vi "Get Device Reference.vi"(11 "VeriStand Framework in":refnum<class "VeriStand DSF.lvclass">=refnum) -> (2 "Device Item Ref":T1=18446744073709551615 format="%.0x", 3 "VeriStand Framework out":refnum<class "VeriStand DSF.lvclass">)   [LabVIEW 2017, in "DSF Engine.lvlib" / "VeriStand DSF.lvclass"]
uses:
  VeriStand DSF.lvclass
  <vilib>/NI Veristand/Custom Device API/Custom Device Item Ref.ctl
  VeriStand DSF.lvclass/VeriStand DSF.ctl
  <vilib>/NI Veristand/Custom Device API/Custom Device API.lvlib
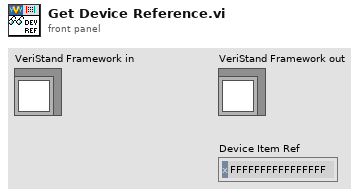
[diagram p1: front panel]
types:
  T1 = typedef "Custom Device API.lvlib/Custom Device Item Ref.ctl" = u64
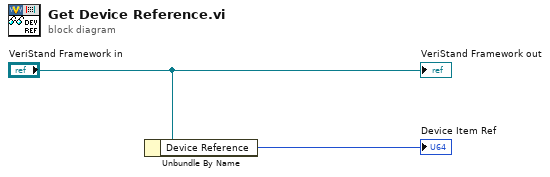
[diagram p0: block diagram]
diagram:
  n1 = Unbundle By Name("VeriStand Framework in") -> ("Device Reference"=→"Device Item Ref":T1)
  "VeriStand Framework out" <- "VeriStand Framework in"
